vi "Insert End Step.vi"(0 "VISA resource name":refnum<visa-resource-name>, 1 "Unit Address (1)":i16=1, 2 "End Step Action (2: All Off)":u16(ring)=2 items=["Hold", "Control Off", "All Off", "Idle"], 5 "Current Step Number (1)":i16=1, 7 "Channel 1 Idle Set Point (75.0)":dbl=75.0 format="%.2f", 9 "Channel 2 Idle Set Point (75.0)":dbl=75.0 format="%.2f", 11 "error in (no error)":errorcluster {"code" format="%.0x"}) -> (4 "VISA resource name out":refnum<visa-resource-name>, 15 "error out":errorcluster {"code" format="%.0x"})   [LabVIEW 2010]
doc: "This VI sets the End Step."
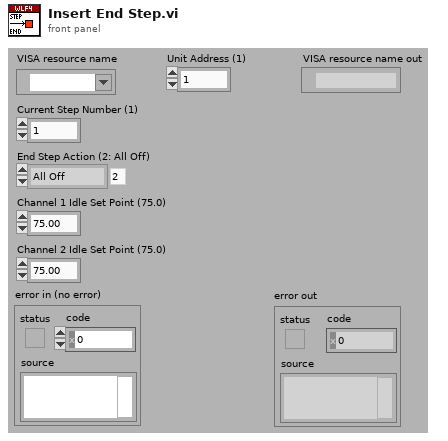
[diagram p1: front panel]
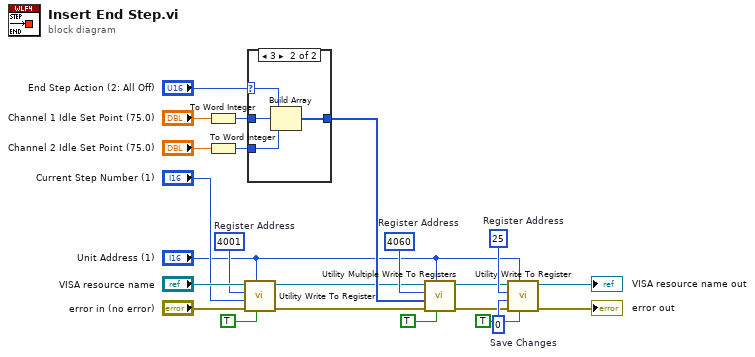
[diagram p0: block diagram]
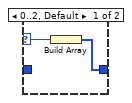
[diagram p2: hidden frame]
diagram:
  w19 = u16 4060  # Register Address
  w20 = i16 0  # Save Changes
  w21 = u16 25  # Register Address
  w7 = u16 4001  # Register Address
  n1 = To Word Integer(number="Channel 1 Idle Set Point (75.0)") -> (16bit integer=w13:i16)
  n2 = To Word Integer(number="Channel 2 Idle Set Point (75.0)") -> (16bit integer=w12:i16)
  n3 = call "Utility Write To Register.vi"("Direct Action?"=TRUE, "Unit Address (1)"="Unit Address (1)", "error in (no error)"="error in (no error)", "Data (0)"="Current Step Number (1)", "Register Address (0)"=w7, "VISA resource name"="VISA resource name") -> ("error out"=w5:errorcluster, "VISA resource name out"=w4:refnum<visa-resource-name>)  [unwired: 4 in]
  n4 = case shown="3" "End Step Action (2: All Off)" {
    selector: "End Step Action (2: All Off)" -> [w25 w29]
    tunnel: w13 -> [_ w28]
    tunnel: w12 -> [_ w27]
    tunnel: [w24 w26] -> w11
    frame 0..2, Default {
      n5 = Build Array(w25) -> (w24:u16[])
    }
    frame 3 {
      n6 = Build Array(w29, w28, w27) -> (w26:u16[])
    }
  }
  n7 = call "Utility Multiple Write To Registers.vi"("Direct Action?"=TRUE, "Unit Address (1)"="Unit Address (1)", "error in (no error)"=w5, "Array Of Data"=w11, "Register Address (0)"=w19, "VISA resource name"=w4) -> ("error out"=w18:errorcluster, "VISA resource name out"=w17:refnum<visa-resource-name>)  [unwired: 4 in]
  n8 = call "Utility Write To Register.vi"("Direct Action?"=TRUE, "Unit Address (1)"="Unit Address (1)", "error in (no error)"=w18, "Data (0)"=w20, "Register Address (0)"=w21, "VISA resource name"=w17) -> ("error out"=→"error out":errorcluster, "VISA resource name out"=→"VISA resource name out":refnum<visa-resource-name>)  [unwired: 4 in]
